vi "prepare image for 2nd mom analysis.vi"(8 "error in (no error)":errorcluster, 11 "Image in":T1) -> (0 "error out":errorcluster, 3 "Image out":T1)   [LabVIEW 2013]
uses:
  IMAQ Image.ctl
  NI_Vision_Development_Module.lvlib
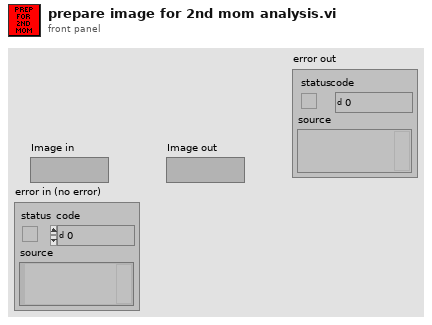
[diagram p1: front panel]
types:
  T1 = typedef "IMAQ Image.ctl" = refnum<image>
  T2 = typedef "Image Type" = u32
  T3 = typedef "ROI Descriptor" = cluster{"Global Rectangle":i32[], "Contours":cluster{"ID":enum32{"External", "Internal"}, "Type":u32, "Coordinates":i32[]}[]}
  T4 = cluster{"histogram":u32[], "Minimal Value":sgl, "Maximal Value":sgl, "Starting Value":sgl, "Interval Width":sgl, "Mean Value":sgl, "Standard  Variation":sgl, "Area (pixels)":i32}
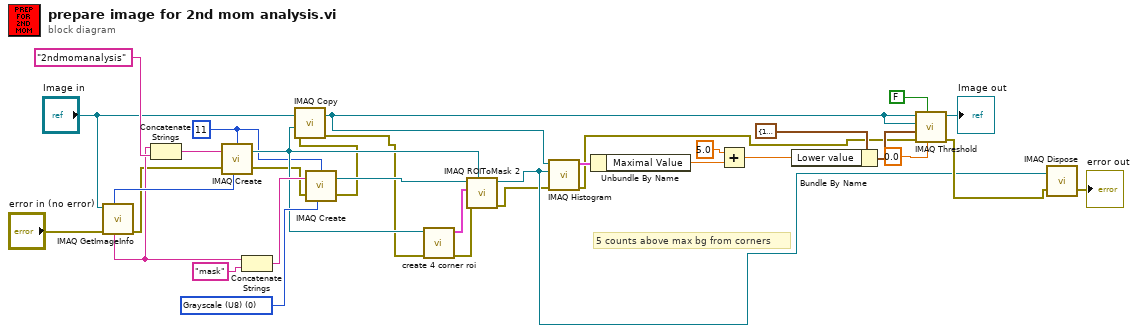
[diagram p0: block diagram]
diagram:
  w28 = T2 0 items=["Grayscale (U8)", "Grayscale (I16)", "Grayscale (SGL)", "Complex (CSG)", "RGB (U32)", "HSL (U32)", "RGB (U64)", "Grayscale (U16)"] ("Image Type")
  w1 = 11 ("Border Size")
  # "5 counts above max bg from corners"
  n1 = call "IMAQ GetImageInfo"("error in (no error)"="error in (no error)", "Image"="Image in") -> ("error out"=w10:errorcluster, "Image Name"=w13:string, "Image Type"=w14:T2)  [unwired: 2 in, 5 out]
  n2 = Concatenate Strings(w13, "2ndmomanalysis" ("Image Name")) -> (w18:string)
  n3 = call "IMAQ Create"("Border Size"=w1, "Image Name"=w18, "Image Type"=w14, "error in (no error)"=w10) -> ("New Image"=w16:T1, "error out"=w9:errorcluster)  [unwired: 1 in]
  n4 = Concatenate Strings(w13, "mask" ("Image Name")) -> (w27:string)
  n5 = call "IMAQ Create"("Border Size"=w1, "Image Name"=w27, "Image Type"=w28, "error in (no error)"=w9) -> ("New Image"=w29:T1, "error out"=w8:errorcluster)  [unwired: 1 in]
  n6 = call "IMAQ Copy"("error in (no error)"=w8, "Image Dst"=w16, "Image Src"="Image in") -> ("error out"=w7:errorcluster, "Image Dst Out"=w31:T1)  [unwired: 3 in]
  n7 = call "create 4 corner roi.vi"("error in (no error)"=w7, "Refnum in"=w16) -> ("error out"=w6:errorcluster, "ROI Descriptor"=w30:T3)  [unwired: 8 in]
  n8 = call "IMAQ ROIToMask 2"("Image Model"=w16, "error in (no error)"=w6, "ROI Descriptor"=w30, "Image"=w29) -> ("error out"=w5:errorcluster, "Image Out"=w11:T1)  [unwired: 5 in, 1 out]
  n9 = call "IMAQ Histogram"("error in (no error)"=w5, "Image Mask"=w11, "Image"=w31) -> ("error out"=w4:errorcluster, "Histogram Report"=w24:T4)  [unwired: 7 in]
  n10 = Unbundle By Name(w24) -> ("Maximal Value"=w25:sgl)
  n11 = Add(x=sgl 5.0, y=w25) -> (x+y=w32:sgl)
  n12 = Bundle By Name(cluster=cluster{"Lower value":sgl, "Upper value":sgl} {"Lower value"=100.0, "Upper value"=9999999.0} ("Range"), "Lower value"=w32) -> (w22:cluster{"Lower value":sgl, "Upper value":sgl})
  n13 = call "IMAQ Threshold"("Replace Value"=sgl 0.0, "Keep/Replace Value (Replace)"=FALSE, "error in (no error)"=w4, "Range"=w22, "Image Dst"=w31, "Image Src"=w31) -> ("error out"=w12:errorcluster, "Image Dst Out"=→"Image out":T1)  [unwired: 4 in]
  n14 = call "IMAQ Dispose"("Image"=w11, "error in (no error)"=w12) -> ("error out"=→"error out":errorcluster)  [unwired: 4 in]
